vi "Log.vi"(7 "Level":T1, 8 "error in":errorcluster, 9 "Error to Log":errorcluster, 10 "Message":string, 11 "Logger in":refnum<class "Logger.lvclass">) -> (0 "error out":errorcluster, 3 "Logger out":refnum<class "Logger.lvclass">)   [LabVIEW 2020, in "hse-logger.lvlib" / "Logger.lvclass"]
doc: "Creates a ``LogRecord`` with the specified level, message and error-cluster, und passes it to the registered ``Handlers``.\n\n____\nHAMPEL SOFTWARE ENGINEERING v2.0.6 (2021-04-15 11:38)"
uses:
  Logger.lvclass
  LogLevel.ctl
  Logger.lvclass/Logger.ctl
  <vilib>/Utility/error.llb/Error Cluster From Error Code.vi
  <vilib>/ErrorRing/Error Ring.xnode
  Handler/Handler.lvclass
  LogRecord/LogRecord.lvclass
  hse-logger.lvlib
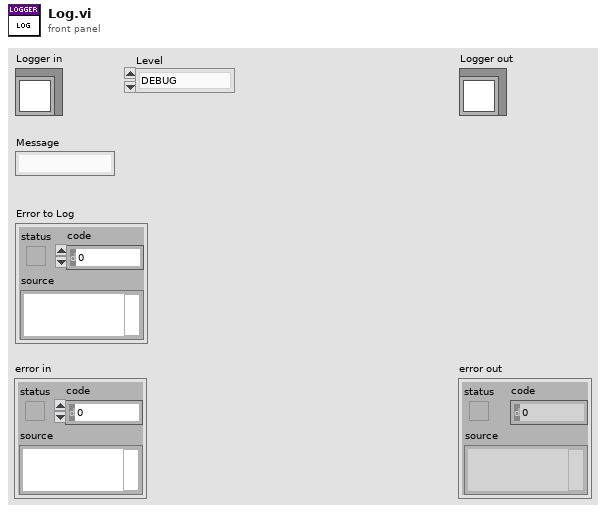
[diagram p1: front panel]
types:
  T1 = typedef "hse-logger.lvlib/LogLevel.ctl" = enum16{"DEBUG", "INFO", "WARNING", "ERROR", "CRITICAL"}
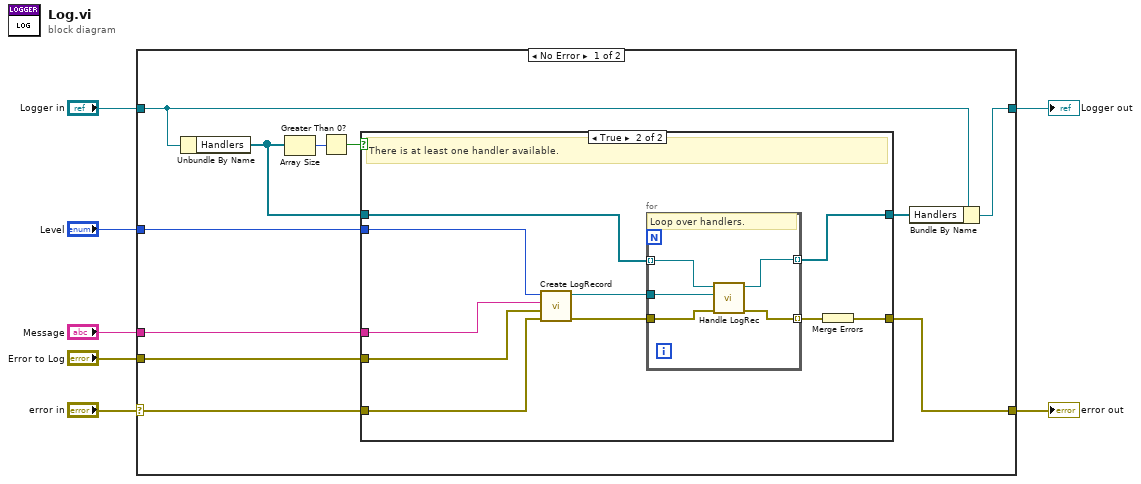
[diagram p0: block diagram]
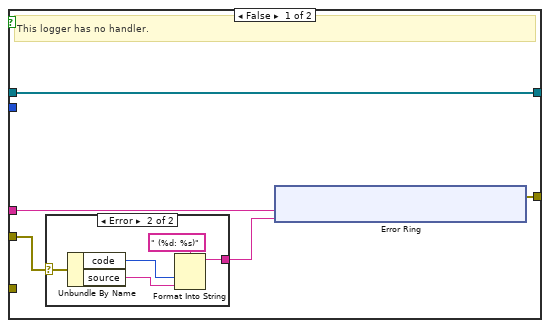
[diagram p2: hidden frame]
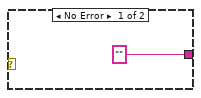
[diagram p3: hidden frame]
diagram:
  n1 = case shown="No Error" "error in" {
    selector: "error in" -> [w11 w54]
    tunnel: [w16 w54] -> w6
    tunnel: [w8 w53] -> w4
    tunnel: "Logger in" -> [w9 w53]
    tunnel: "Level" -> [w14 _]
    tunnel: "Message" -> [w13 _]
    tunnel: "Error to Log" -> [w12 _]
    frame No Error {
      n2 = Unbundle By Name(w9) -> ("Handlers"=w15:refnum<class "Handler.lvclass">[])
      n3 = Array Size(array=w15) -> (size(s)=w18:i32)
      n4 = Greater Than 0?(x=w18) -> (x > 0?=w17:bool)
      n5 = case shown="True" w17 {
        tunnel: [w22 w45] -> w16
        tunnel: w15 -> [w19 w46]
        tunnel: w14 -> [_ w39]
        tunnel: w13 -> [w20 w42]
        tunnel: w12 -> [w23 w41]
        tunnel: w11 -> [_ w40]
        tunnel: [w19 w38] -> w10
        frame False {
          # "This logger has no handler."
          n6 = case shown="Error" w23 {
            selector: w23 -> [_ w37]
            tunnel: ["" w36] -> w21
            frame No Error {
            }
            frame Error {
              n7 = Unbundle By Name(w37) -> ("code"=w34:i32, "source"=w35:string)
              n8 = Format Into String(format string=" (%d: %s)", w34, w35) -> (resulting string=w36:string)  [unwired: 2 in, 1 out]
            }
          }
          n9 = xnode "Error Ring"("parameter 0"=w20, "parameter 1"=w21) -> ("error out"=w22:errorcluster)
        }
        frame True {
          # "There is at least one handler available."
          n10 = call "Create LogRecord.vi"("error in"=w40, "Error to Log"=w41, "Message"=w42, "Level"=w39) -> ("error out"=w43:errorcluster, "LogRecord out"=w44:refnum<class "LogRecord.lvclass">)  [unwired: 6 in]
          n11 = for {
            tunnel: w46 -> [w52] mode=indexing
            tunnel: w44 -> [w51]
            tunnel: w43 -> [w50]
            tunnel: [w49] -> w47 mode=indexing
            tunnel: [w48] -> w38 mode=indexing
            # "Loop over handlers."
            n12 = call-dynamic "Handle LogRec.vi"("error in"=w50, "LogRecord"=w51, "Handler in"=w52) -> ("error out"=w49:errorcluster, "Handler out"=w48:refnum<class "Handler.lvclass">)  [unwired: 7 in]
          }
          n13 = Merge Errors(w47) -> (w45:errorcluster)
        }
      }
      n14 = Bundle By Name(cluster=w9, "Handlers"=w10) -> (w8:refnum<class "Logger.lvclass">)
    }
    frame Error {
    }
  }
  "error out" <- w6
  "Logger out" <- w4
